vi "TrendsD02.vi"() -> ()   [LabVIEW 2019, in "D02.lvlib"]
uses:
  D02.lvlib
  <vilib>/measure/mamon.llb/Trigger Detection for 1 Channel.vi
  <vilib>/measure/NI_MAPro.lvlib
panel:
  out "No Change":bool
  out "Sudden Change":bool
  out "Decrease":bool
  out "Increase":bool
  out "Previous  ES":dbl
  out "Present  Speed":dbl
  out "Present Error":dbl format="%#.2g"
  out "Previous Error":dbl
  out "Previous  Speed":dbl
  out "Previous PW":dbl caption="Control Information"
  out "Pulse Trends":waveform(i16)[](graph) caption="Waveform Chart - Dark"
  in  "Close":bool
  out "disc name":string="Disc 02 Trends"
  out "dsgs":string="DSGS"
  out "Speed Trend":waveform(dbl)(graph) caption="Waveform Chart - Dark"
  out "Average Trend":waveform(dbl)[](graph) caption="Waveform Chart - Dark"
  out "Live Trend":waveform(dbl)[](graph) caption="Waveform Chart - Dark"
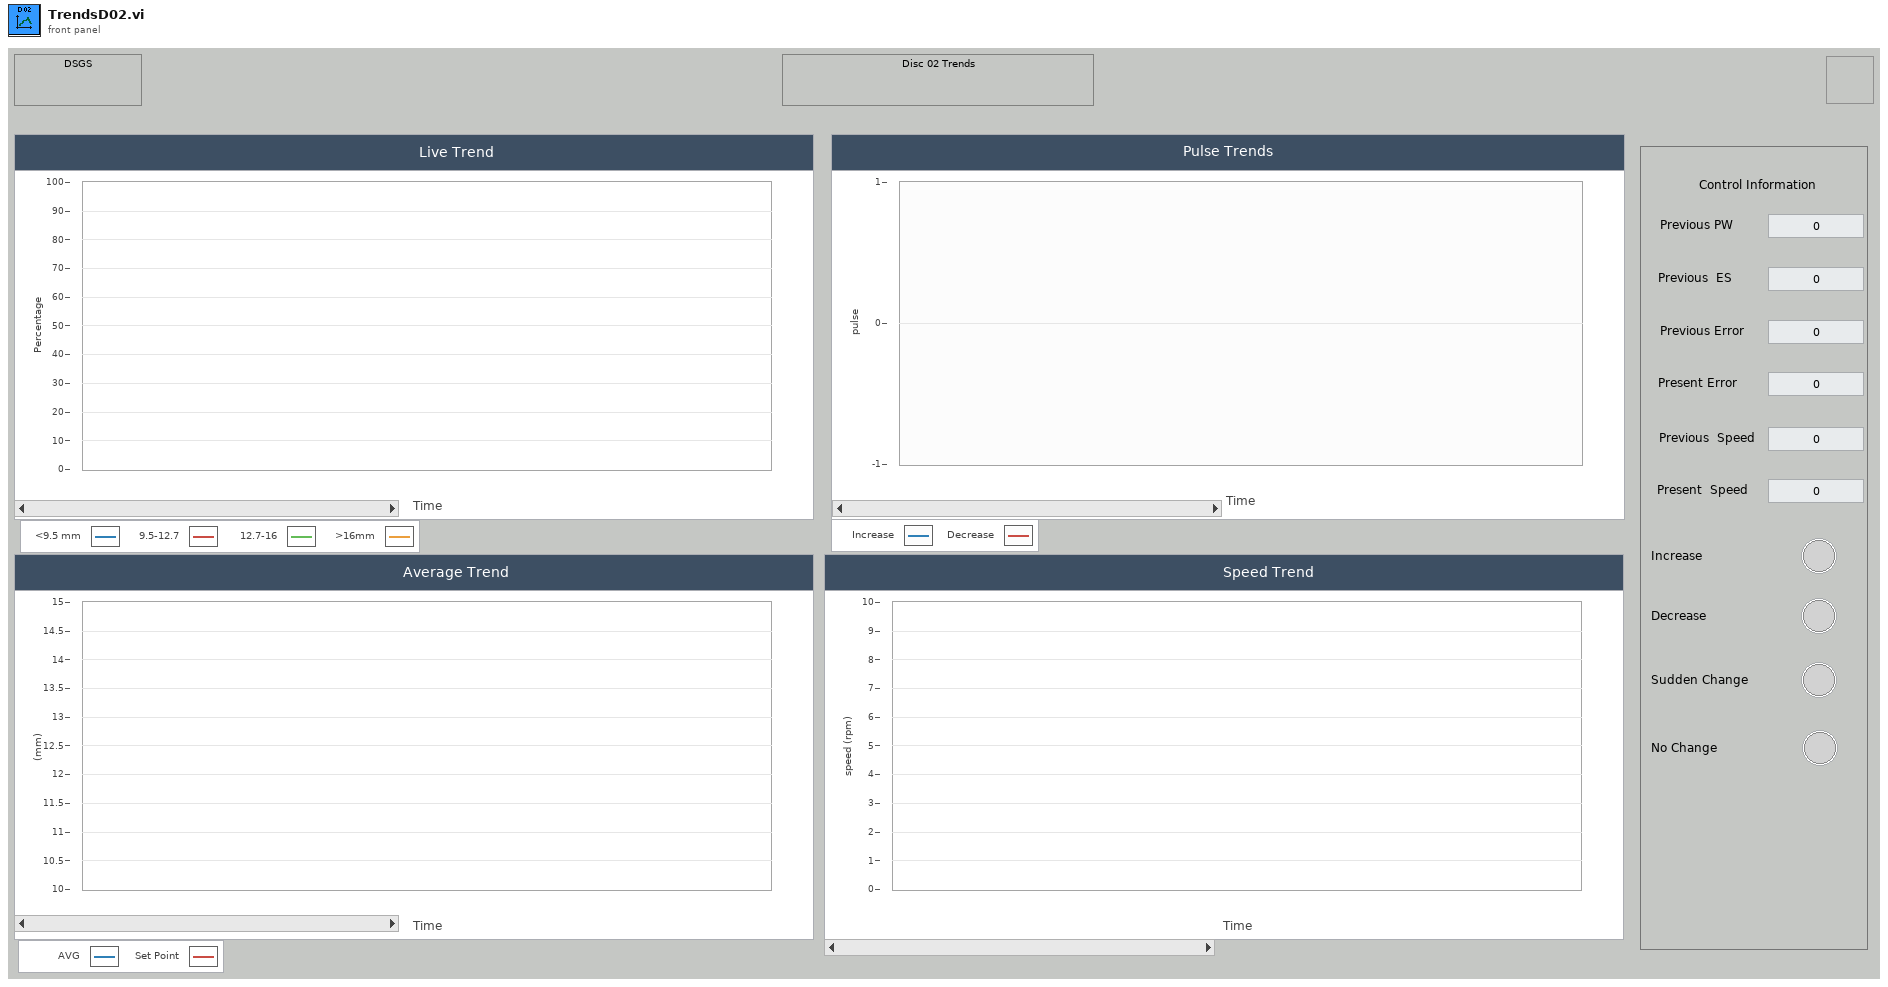
[diagram p1: front panel]
types:
  T1 = cluster{"decrease D02":bool, "increase D02":bool, "no change D02":bool, "sudden change D02":bool, "last error 02":dbl, "previous speed D02":dbl, "pulse width D02":dbl, "slope D02":dbl}
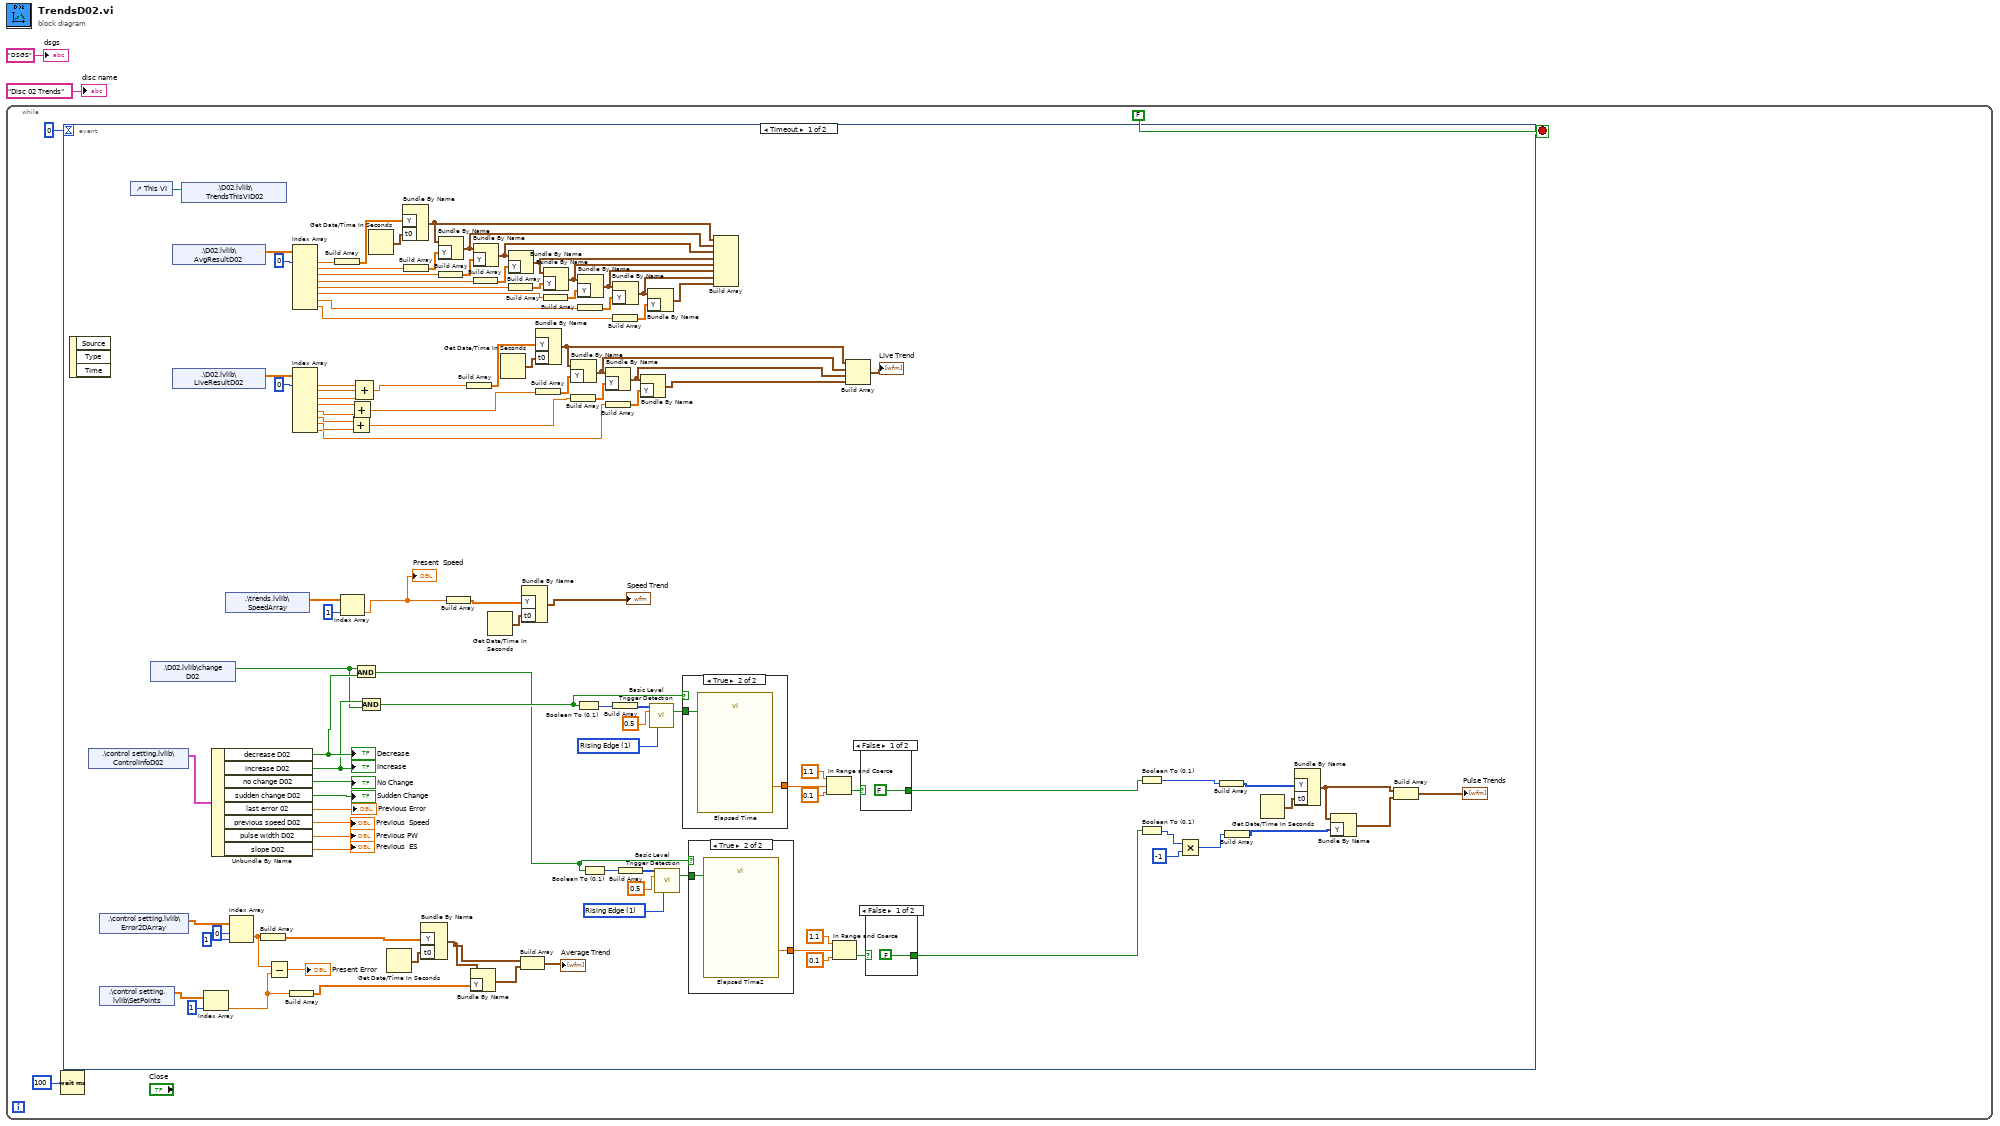
[diagram p0: block diagram]
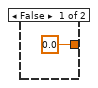
[diagram p2: hidden frame]
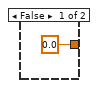
[diagram p4: hidden frame]
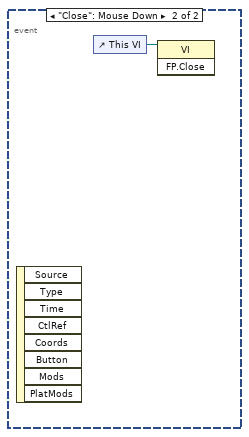
[diagram p6: hidden frame]
diagram:
  n1 = while {
    stop <- FALSE stop-if-true
    n2 = Wait (ms)(milliseconds to wait=u32 100) -> ()  [unwired: 1 out]
    n3 = event shown="[0] Timeout" {
      selector: _ -> [_ _]
      dyn-events: _ -> [_ _]
      timeout: 0 -> [_ _]
      event Timeout {
        w36 = u16 1 items=["Falling Edge", "Rising Edge"] ("trigger slope")
        w40 = u16 1 items=["Falling Edge", "Rising Edge"] ("trigger slope")
        n4 = event-data() -> ()  [unwired: 1 in, 3 out]
        n5 = shared-variable ".\\control setting.lvlib\\ControlInfoD02"() -> (w63:T1)  [unwired: 1 in, 1 out]
        n6 = shared-variable ".\\control setting.lvlib\\Error2DArray"() -> (w57:dbl[][])  [unwired: 1 in, 1 out]
        n7 = shared-variable ".\\control setting.lvlib\\SetPoints"() -> (w54:dbl[])  [unwired: 1 in, 1 out]
        n8 = control-ref of="This VI"() -> (w79:refnum<vi>)
        n9 = shared-variable ".\\D02.lvlib\\change D02"() -> (w48:bool)  [unwired: 1 in, 1 out]
        n10 = shared-variable ".\\D02.lvlib\\AvgResultD02"() -> (w85:dbl[])  [unwired: 1 in, 1 out]
        n11 = shared-variable ".\\D02.lvlib\\LiveResultD02"() -> (w118:dbl[])  [unwired: 1 in, 1 out]
        n12 = shared-variable ".\\D02.lvlib\\TrendsThisVID02"(w79) -> ()  [unwired: 1 in, 1 out]
        n13 = Index Array(array=w54, index=1) -> (element=w10:dbl)
        n14 = Unbundle By Name(w63) -> ("decrease D02"=w50:bool, "increase D02"=w49:bool, "no change D02"=→"No Change":bool, "sudden change D02"=→"Sudden Change":bool, "last error 02"=→"Previous Error":dbl, "previous speed D02"=→"Previous  Speed":dbl, "pulse width D02"=→"Previous PW":dbl, "slope D02"=→"Previous  ES":dbl)
        "Increase" <- w49
        "Decrease" <- w50
        n15 = shared-variable ".\\trends.lvlib\\SpeedArray"() -> (w68:dbl[])  [unwired: 1 in, 1 out]
        n16 = Index Array(array=w57, index (row)=0, index (col)=1 ("disabled index (col)")) -> (element=w23:dbl)
        n17 = Build Array(w23) -> (w25:dbl[])
        n18 = Subtract(x=w23, y=w10) -> (x-y=→"Present Error":dbl)
        n19 = Build Array(w10) -> (w9:dbl[])
        n20 = Index Array(array=w85, index #1=0 ("index")) -> (element #1=w95:dbl, element #2=w96:dbl, element #3=w98:dbl, element #4=w100:dbl, element #5=w101:dbl, element #6=w103:dbl, element #7=w105:dbl, element #8=w84:dbl)  [unwired: 7 in]
        n21 = Index Array(array=w118, index #1=0 ("index")) -> (element #1=w22:dbl, element #2=w21:dbl, element #3=w20:dbl, element #4=w18:dbl, element #5=w17:dbl, element #6=w16:dbl, element #7=w15:dbl, element #8=w12:dbl)  [unwired: 7 in]
        n22 = Build Array(w95) -> (w106:dbl[])
        n23 = Index Array(array=w68, index=1) -> (element=w51:dbl)
        "Present  Speed" <- w51
        n24 = Add(x=w16, y=w15) -> (x+y=w13:dbl)
        n25 = Add(x=w18, y=w17) -> (x+y=w14:dbl)
        n26 = And(x=w48, y=w50) -> (x .and. y?=w28:bool)
        n27 = Compound Arithmetic op=ADD(w22, w21, w20) -> (w19:dbl)
        n28 = And(x=w49, y=w48) -> (x .and. y?=w38:bool)
        n29 = Get Date/Time In Seconds() -> (seconds since 1Jan1904=w88:timestamp)
        n30 = Get Date/Time In Seconds() -> (seconds since 1Jan1904=w24:timestamp)
        n31 = Bundle By Name("Y"=w106, "t0"=w88) -> (w94:waveform(dbl))  [unwired: 1 in]
        n32 = Build Array(w96) -> (w97:dbl[])
        n33 = Bundle By Name("Y"=w25, "t0"=w24) -> (w8:waveform(dbl))  [unwired: 1 in]
        n34 = Bundle By Name(cluster=w94, "Y"=w97) -> (w93:waveform(dbl))
        n35 = Build Array(w98) -> (w99:dbl[])
        n36 = Build Array(w51) -> (w66:dbl[])
        n37 = Build Array(w19) -> (w108:dbl[])
        n38 = Bundle By Name(cluster=w8, "Y"=w9) -> (w7:waveform(dbl))
        n39 = Bundle By Name(cluster=w93, "Y"=w99) -> (w92:waveform(dbl))
        n40 = Build Array(w100) -> (w87:dbl[])
        n41 = Get Date/Time In Seconds() -> (seconds since 1Jan1904=w65:timestamp)
        n42 = Get Date/Time In Seconds() -> (seconds since 1Jan1904=w115:timestamp)
        n43 = Bundle By Name(cluster=w92, "Y"=w87) -> (w91:waveform(dbl))
        n44 = Build Array(w101) -> (w102:dbl[])
        n45 = Build Array(w8, w7) -> (→"Average Trend":waveform(dbl)[])
        n46 = Bundle By Name("Y"=w66, "t0"=w65) -> (→"Speed Trend":waveform(dbl))  [unwired: 1 in]
        n47 = Bundle By Name("Y"=w108, "t0"=w115) -> (w111:waveform(dbl))  [unwired: 1 in]
        n48 = Build Array(w14) -> (w110:dbl[])
        n49 = Bundle By Name(cluster=w91, "Y"=w102) -> (w90:waveform(dbl))
        n50 = Build Array(w103) -> (w104:dbl[])
        n51 = Bundle By Name(cluster=w111, "Y"=w110) -> (w112:waveform(dbl))
        n52 = Build Array(w13) -> (w109:dbl[])
        n53 = Boolean To (0,1)(Boolean=w38) -> (0, 1=w43:i16)
        n54 = Bundle By Name(cluster=w90, "Y"=w104) -> (w89:waveform(dbl))
        n55 = Build Array(w105) -> (w107:dbl[])
        n56 = Boolean To (0,1)(Boolean=w28) -> (0, 1=w33:i16)
        n57 = Bundle By Name(cluster=w112, "Y"=w109) -> (w113:waveform(dbl))
        n58 = Build Array(w12) -> (w116:dbl[])
        n59 = Bundle By Name(cluster=w89, "Y"=w107) -> (w81:waveform(dbl))
        n60 = Build Array(w84) -> (w83:dbl[])
        n61 = Build Array(w43) -> (w42:i16[])
        n62 = Build Array(w33) -> (w34:i16[])
        n63 = Bundle By Name(cluster=w113, "Y"=w116) -> (w114:waveform(dbl))
        n64 = Bundle By Name(cluster=w81, "Y"=w83) -> (w82:waveform(dbl))
        n65 = call-poly <vilib>:"Basic Level Trigger Detection.vi"("signal in"=w42, "level"=0.5, "trigger slope"=w40) -> ("trigger detected?"=w39:bool)  [unwired: 10 in, 2 out]
        n66 = call-poly <vilib>:"Basic Level Trigger Detection.vi"("signal in"=w34, "level"=0.5, "trigger slope"=w36) -> ("trigger detected?"=w37:bool)  [unwired: 10 in, 2 out]
        n67 = case shown="True" w38 {
          tunnel: [0.0 ("Elapsed Time (s)") w125] -> w47
          tunnel: w39 -> [_ w126]
          frame False {
          }
          frame True {
            n68 = call "Elapsed Time"("Reset"=w126) -> ("Elapsed Time (s)"=w125:dbl)  [unwired: 11 in, 7 out]
          }
        }
        n69 = case shown="True" w28 {
          tunnel: [0.0 ("Elapsed Time (s)") w120] -> w29
          tunnel: w37 -> [_ w121]
          frame False {
          }
          frame True {
            n70 = call "Elapsed Time2"("Reset"=w121) -> ("Elapsed Time (s)"=w120:dbl)  [unwired: 11 in, 7 out]
          }
        }
        n71 = Build Array(w94, w93, w92, w91, w90, w89, w81, w82) -> ()  [unwired: 1 out]
        n72 = In Range and Coerce(upper limit=1.1, x=w47, lower limit=0.1) -> (In Range?=w44:bool)  [unwired: 1 out]
        n73 = In Range and Coerce(upper limit=1.1, x=w29, lower limit=0.1) -> (In Range?=w32:bool)  [unwired: 1 out]
        n74 = Build Array(w111, w112, w113, w114) -> (→"Live Trend":waveform(dbl)[])
        n75 = case shown="False" w44 {
          selector: w44 -> [_ w128]
          tunnel: [FALSE w128] -> w27
          frame False {
          }
          frame True {
          }
        }
        n76 = case shown="False" w32 {
          selector: w32 -> [_ w123]
          tunnel: [FALSE w123] -> w26
          frame False {
          }
          frame True {
          }
        }
        n77 = Boolean To (0,1)(Boolean=w27) -> (0, 1=w76:i16)
        n78 = Boolean To (0,1)(Boolean=w26) -> (0, 1=w72:i16)
        n79 = Multiply(x=w72, y=i16 -1 ("0, 1")) -> (x*y=w70:i16)
        n80 = Build Array(w76) -> (w77:i16[])
        n81 = Build Array(w70) -> (w75:i16[])
        n82 = Get Date/Time In Seconds() -> (seconds since 1Jan1904=w78:timestamp)
        n83 = Bundle By Name("Y"=w77, "t0"=w78) -> (w74:waveform(i16))  [unwired: 1 in]
        n84 = Bundle By Name(cluster=w74, "Y"=w75) -> (w73:waveform(i16))
        n85 = Build Array(w74, w73) -> (→"Pulse Trends":waveform(i16)[])
      }
      event "Close": Mouse Down {
        n86 = event-data() -> ()  [unwired: 1 in, 8 out]
        n87 = control-ref of="This VI"() -> (w129:refnum<vi>)
        n88 = invoke class="VI" method="FP.Close"(reference=w129) -> ()  [unwired: 2 in, 3 out]
      }
    }
  }
  "dsgs" <- "DSGS" ("dsgs")
  "disc name" <- "Disc 02 Trends" ("disc name")
